vi "PLC.Dial800._TEST Read Bool Value, Timing Check.vi"() -> ()   [LabVIEW 2018]
uses:
  <vilib>/KATE/Time/Time Utils.lvlib
panel:
  in  "wait for updated value (T)":bool
  out "Error Out":errorcluster
  in  "stop":bool
  out "Duration(s)":dbl
  out "timestamp":timestamp
  out "Boolean":bool
  in  "URL":string
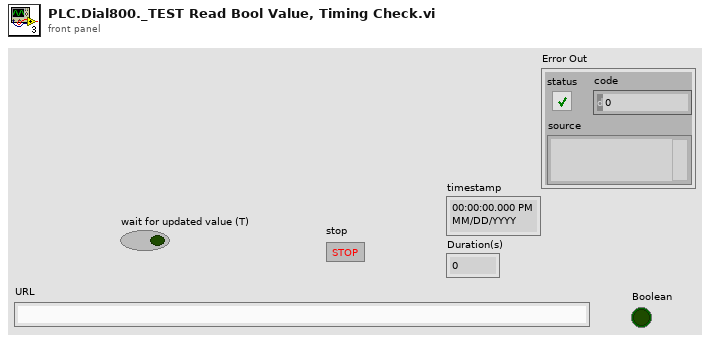
[diagram p1: front panel]
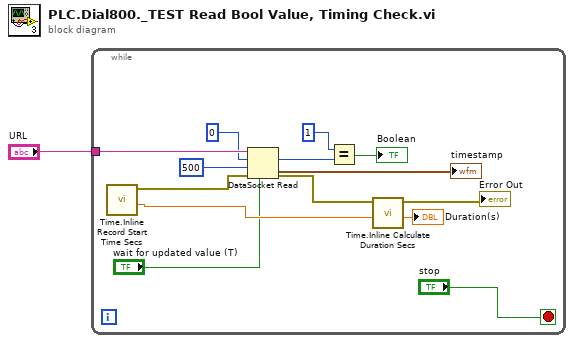
[diagram p0: block diagram]
diagram:
  n1 = while {
    tunnel: "URL" -> [w15]
    stop <- "stop" stop-if-true
    n2 = call <vilib>:"Time.Inline Record Start Time Secs.vi"() -> ("Start(s)"=w6:dbl, "Error Out Upper"=w14:errorcluster)  [unwired: 9 in, 1 out]
    n3 = DataSocket Read(6:"wait for updated value (T)", 8:w14, 9:500 ("ms timeout (10000)"), 10:0, 11:w15) -> (0:w7:errorcluster, 2:w12:i32, 4:→"timestamp":timestamp)  [unwired: 4 out]
    n4 = Equal?(x=1, y=w12) -> (x = y?=→"Boolean":bool)
    n5 = call <vilib>:"Time.Inline Calculate Duration Secs.vi"("Start(Sec)"=w6, "Error In Top"=w7) -> ("Duration(s)"=→"Duration(s)":dbl, "Error Out Top"=→"Error Out":errorcluster)  [unwired: 7 in, 1 out]
  }
